vi "FGV.vi"(7 "Action":T1, 8 "error in (no error)":errorcluster, 10 "IAmGLF To Create DVR":refnum<class "IAmGLF.lvclass">, 11 "IAmEngine":refnum<class "IAmEngine.lvclass">) -> (0 "error out":errorcluster)   [LabVIEW 2024, in "GLF.lvlib" / "DVRHandler.lvlib"]
uses:
  DVRHandler.lvlib
  IAmEngine/IAmEngine.lvclass
  IAmGLF/IAmGLF.lvclass
  Action--enum.ctl
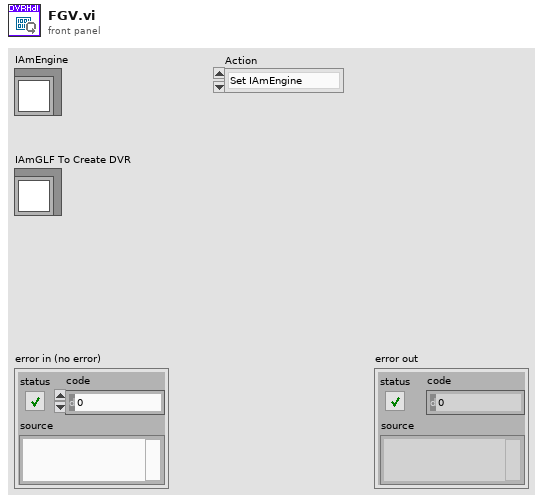
[diagram p1: front panel]
types:
  T1 = typedef "GLF.lvlib/DVRHandler.lvlib/Action--enum.ctl" = enum16{"Set IAmEngine"}
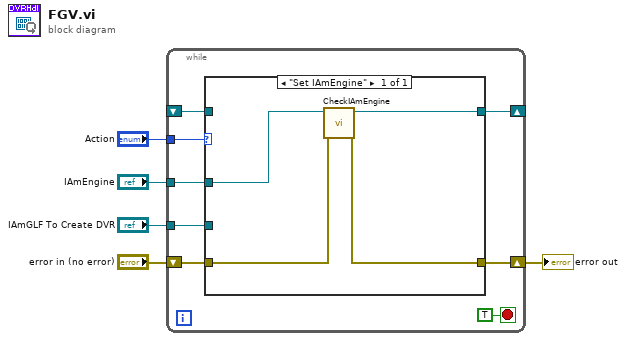
[diagram p0: block diagram]
diagram:
  n1 = while {
    tunnel: "IAmEngine" -> [w13]
    tunnel: "IAmGLF To Create DVR" -> [w11]
    tunnel: "Action" -> [w9]
    shift-right: [w10] -> w2
    shift-left: "error in (no error)" -> [w12]
    shift-right: [w7] -> _
    shift-left: _ -> [w6]
    stop <- TRUE stop-if-true
    n2 = case shown="\"Set IAmEngine\"" w9 {
      tunnel: w13 -> [w17]
      tunnel: w12 -> [w15]
      tunnel: w11 -> [_]
      tunnel: [w14] -> w10
      tunnel: [w16] -> w7
      tunnel: w6 -> [_]
      frame "Set IAmEngine" {
        n3 = call "CheckIAmEngine.vi"("error in (no error)"=w15, "IAmEngine In"=w17) -> ("error out"=w14:errorcluster, "IAmEngine Out"=w16:refnum<class "IAmEngine.lvclass">)  [unwired: 8 in]
      }
    }
  }
  "error out" <- w2
